vi "LV-Solver.vi"(10 "Word List":string[](array[string]), 11 "Word Search Grid":string[][](array[string])) -> (3 "Solutions":T1)   [LabVIEW 2020]
uses:
  support/Letter Index--cluster.ctl
  support/Solutions--map.ctl
panel:
  # "Implement your Word Search challenge solution in this VI. Do not change the connector pane of this VI."
  # "Letters will always be ALL CAPS."
  # "Words will always be ALL CAPS."
  # "The Word Search Grid contains the 2D array of letters in which all words in the Word List appear. Words can appear forwards, backwards, up, down, and diagonally in any direction.\n\nThe Solutions map will contain one entry per item in the Word List. The map elements are:\n\nWord: The word from the Word List.\nLetter Indices: The row/column indices into the Word Search Grid for each letter (in order) in the word."
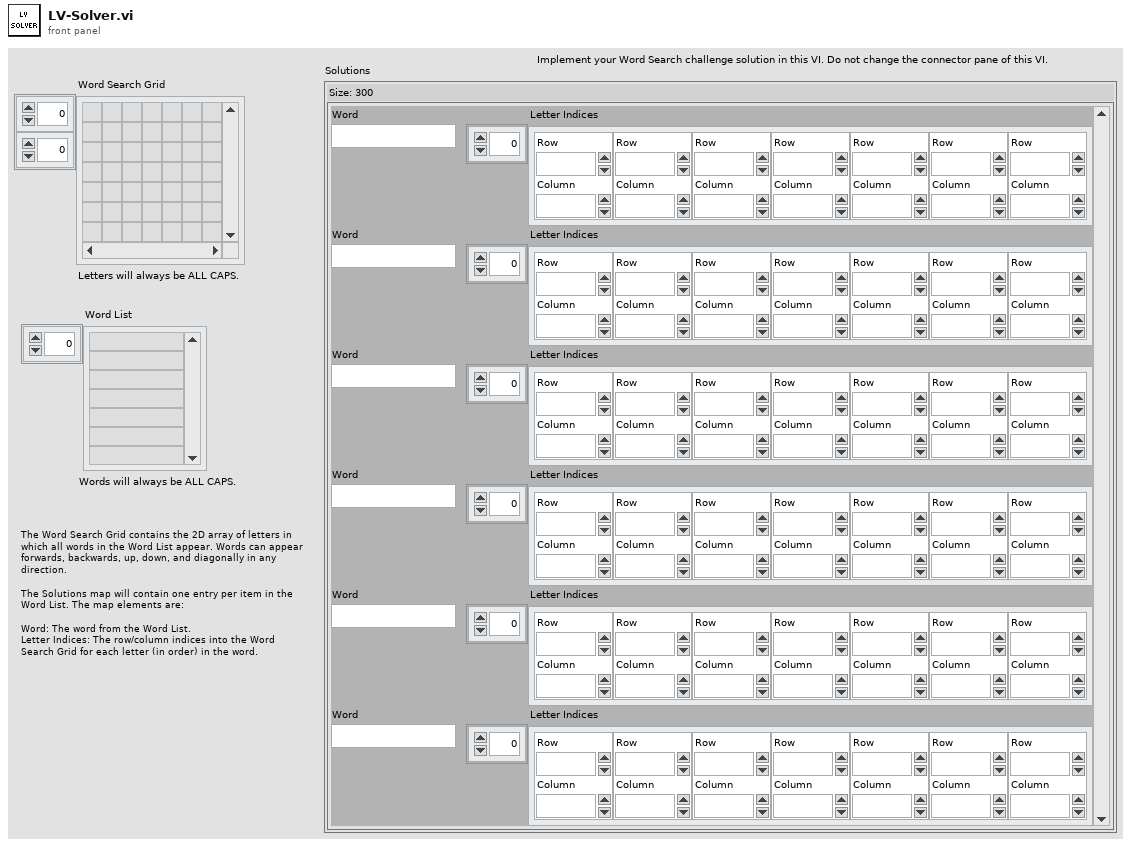
[diagram p1: front panel]
types:
  T1 = typedef "Solutions--map.ctl" = map{string, T2[]}
  T2 = typedef "Letter Index--cluster.ctl" = cluster{"Row":i32, "Column":i32}
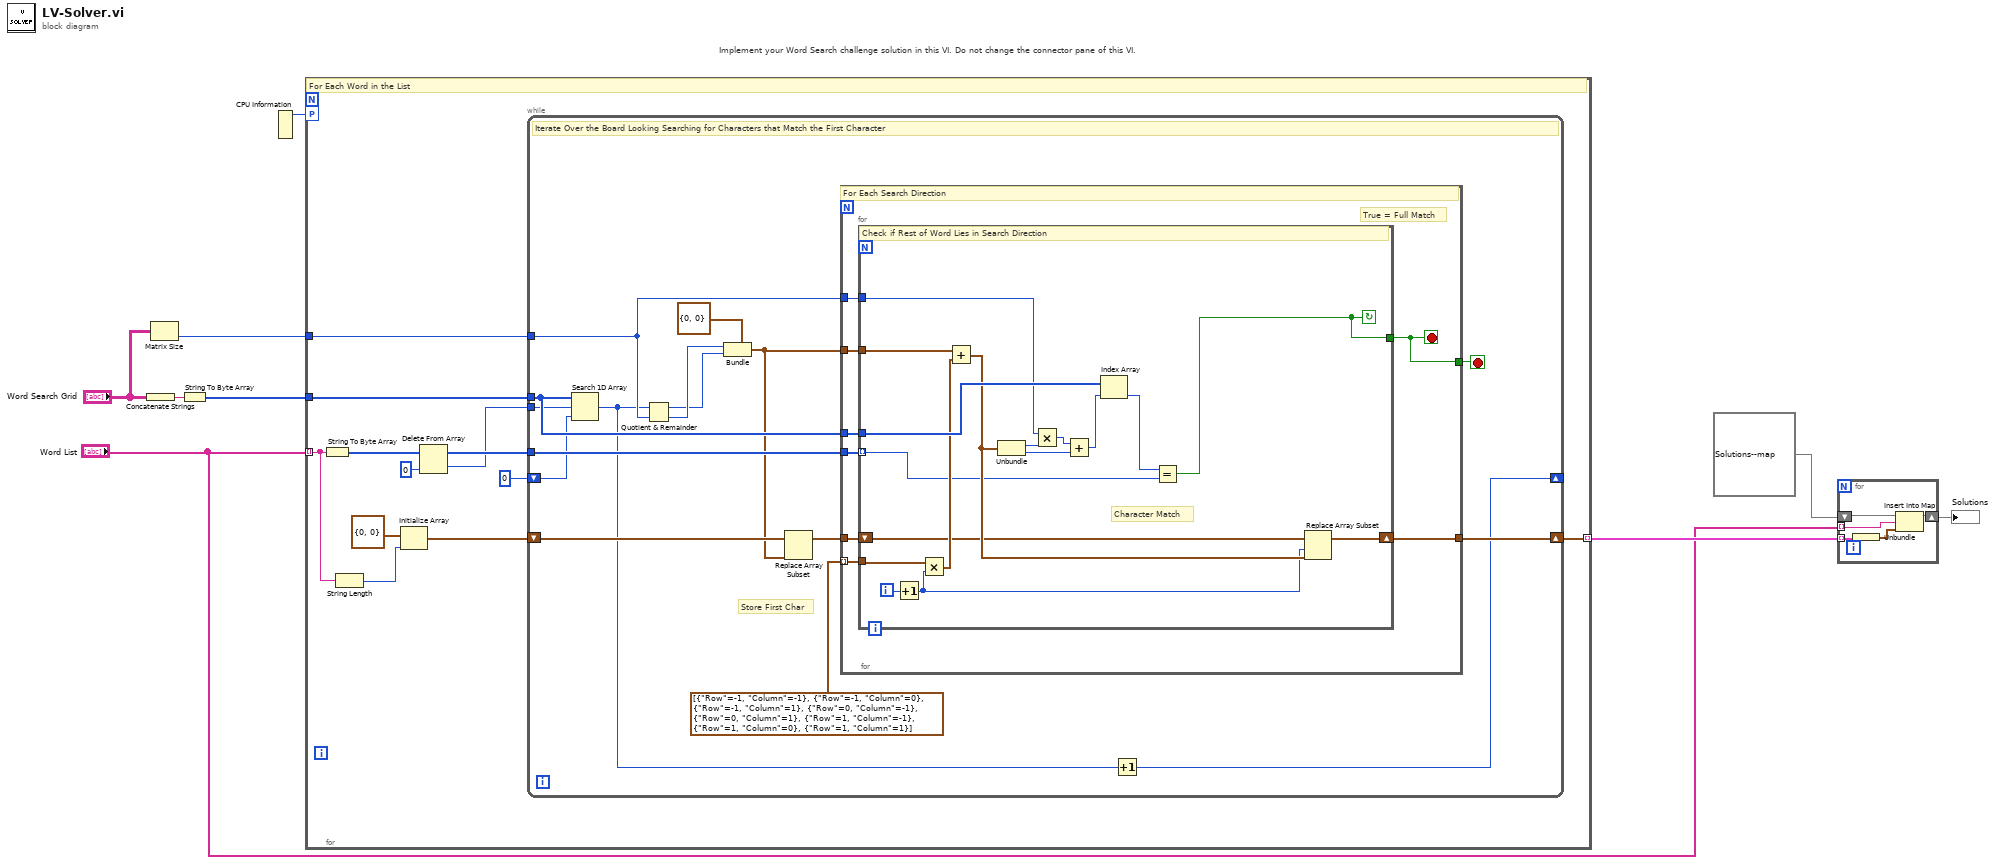
[diagram p0: block diagram]
diagram:
  # "Implement your Word Search challenge solution in this VI. Do not change the connector pane of this VI."
  n1 = Concatenate Strings("Word Search Grid") -> (w9:string)
  n2 = Matrix Size(0:"Word Search Grid") -> (2:w1:i32)  [unwired: 1 out]
  n3 = String To Byte Array(string=w9) -> (unsigned byte array=w3:u8[])
  n4 = CPU Information() -> (4:w6:i32)  [unwired: 3 out]
  n5 = for {
    tunnel: w3 -> [w16]
    tunnel: "Word List" -> [w22] mode=indexing
    tunnel: [w17] -> w8 mode=indexing
    workers-P: w6 -> [_]
    tunnel: w1 -> [w14]
    # "For Each Word in the List"
    n6 = String To Byte Array(string=w22) -> (unsigned byte array=w15:u8[])
    n7 = String Length(string=w22) -> (length=w20:i32)
    n8 = Initialize Array(T2 {"Row"=0, "Column"=0} ("Letter Index"), w20) -> (w19:T2[])
    n9 = Delete From Array(array=w15, index=0) -> (deleted portion=w12:u8, array with subset deleted=w13:u8[])  [unwired: 1 in]
    n10 = while {
      tunnel: w16 -> [w36]
      tunnel: w14 -> [w35]
      tunnel: w13 -> [w34]
      tunnel: w12 -> [w33]
      shift-right: [w37] -> w18
      shift-left: w19 -> [w38]
      shift-right: [w24] -> _
      shift-left: 0 ("start index (0)") -> [w32]
      stop <- w23 stop-if-true
      # "Store First Char"
      # "Iterate Over the Board Looking Searching for Characters that Match the First Character"
      n11 = Search 1D Array(1D array=w36, element=w33, start index (0)=w32) -> (index of element=w25:i32)
      n12 = Quotient & Remainder(x=w25, y=w35) -> (x-y*floor(x/y)=w26:i32, floor(x/y)=w27:i32)
      n13 = Bundle(cluster=T2 {"Row"=0, "Column"=0} ("Letter Index"), "Row"=w27, "Column"=w26) -> (w28:T2)
      n14 = Replace Array Subset(array=w38, new element=w28) -> (w31:T2[])  [unwired: 1 in]
      n15 = for {
        tunnel: w31 -> [w42]
        tunnel: T2[] [{"Row"=-1, "Column"=-1}, {"Row"=-1, "Column"=0}, {"Row"=-1, "Column"=1}, {"Row"=0, "Column"=-1}, {"Row"=0, "Column"=1}, {"Row"=1, "Column"=-1}, {"Row"=1, "Column"=0}, {"Row"=1, "Column"=1}] ("Array") -> [w45] mode=indexing
        tunnel: w36 -> [w46]
        tunnel: w34 -> [w44]
        tunnel: [w43] -> w37
        tunnel: w28 -> [w41]
        tunnel: w35 -> [w40]
        tunnel: [w39] -> w23
        stop <- w39 stop-if-true
        # "True = Full Match"
        # "For Each Search Direction"
        n16 = for {
          tunnel: w46 -> [w63]
          tunnel: w45 -> [w61]
          shift-right: [w55] -> w43
          shift-left: w42 -> [w58]
          tunnel: w44 -> [w57] mode=indexing
          tunnel: [w52] -> w39
          tunnel: w41 -> [w54]
          tunnel: w40 -> [w50]
          i -> [w60]
          stop <- w52 continue-if-true
          # "Character Match"
          # "Check if Rest of Word Lies in Search Direction"
          n17 = Increment(x=w60) -> (x+1=w56:i32)
          n18 = Multiply(x=w61, y=w56) -> (x*y=w59:T2)
          n19 = Add(x=w54, y=w59) -> (x+y=w62:T2)
          n20 = Unbundle(w62) -> ("Row"=w51:i32, "Column"=w48:i32)
          n21 = Multiply(x=w50, y=w51) -> (x*y=w49:i32)
          n22 = Add(x=w49, y=w48) -> (x+y=w47:i32)
          n23 = Index Array(array=w63, index=w47) -> (element=w53:u8)
          n24 = Equal?(x=w53, y=w57) -> (x = y?=w52:bool)
          n25 = Replace Array Subset(array=w58, new element=w62, index=w56) -> (w55:T2[])
        }
      }
      n26 = Increment(x=w25) -> (x+1=w24:i32)
    }
    n27 = Bundle(w18) -> (w17:cluster{T2[]})  [unwired: 1 in]
  }
  n28 = for {
    tunnel: w8 -> [w66] mode=indexing
    shift-right: [w67] -> w4
    shift-left: T1 {} ("Solutions") -> [w68]
    tunnel: "Word List" -> [w65] mode=indexing
    n29 = Unbundle(w66) -> (w64:T2[])
    n30 = Insert Into Map(map in=w68, key=w65, value=w64) -> (map out=w67:T1)  [unwired: 2 out]
  }
  "Solutions" <- w4
